vi "Optimal Angle Calc..vi"(8 "Command Angle":dbl, 9 "Feedback Angle":dbl, 11 "Speed":dbl) -> (0 "Angle":dbl, 3 "Speed":dbl)   [LabVIEW 2018]
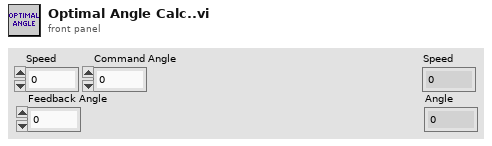
[diagram p1: front panel]
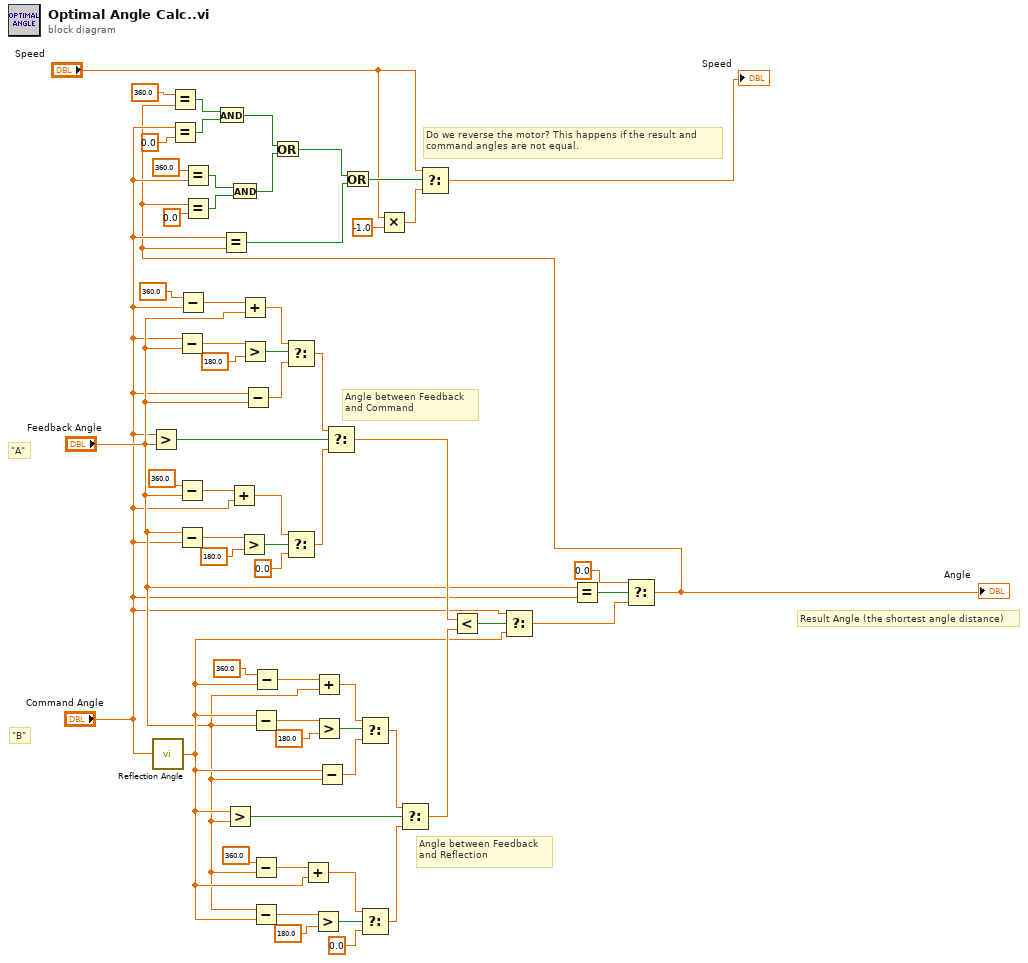
[diagram p0: block diagram]
diagram:
  # "Result Angle (the shortest angle distance)"
  # "Do we reverse the motor? This happens if the result and \ncommand angles are not equal."
  # "Angle between Feedback\nand Reflection"
  # "Angle between Feedback\nand Command"
  # "\"B\""
  # "\"A\""
  n1 = Greater?(x="Command Angle", y="Feedback Angle") -> (0:w61:bool)
  n2 = call "Reflection Angle.vi"("Command Angle"="Command Angle") -> ("Reflection Angle"=w24:dbl)  [unwired: 4 in]
  n3 = Equal?(x="Command Angle", y=0.0) -> (x = y?=w20:bool)
  n4 = Subtract(x="Command Angle", y="Feedback Angle") -> (x-y=w60:dbl)
  n5 = Subtract(x=360.0, y="Feedback Angle") -> (x-y=w48:dbl)
  n6 = Subtract(x="Feedback Angle", y="Command Angle") -> (x-y=w52:dbl)
  n7 = Subtract(x=360.0, y="Command Angle") -> (x-y=w56:dbl)
  n8 = Equal?(x=360.0, y="Command Angle") -> (x = y?=w18:bool)
  n9 = Greater?(x=w24, y="Feedback Angle") -> (0:w44:bool)
  n10 = Add(x=w48, y="Command Angle") -> (x+y=w47:dbl)
  n11 = Greater?(x=w52, y=180.0) -> (0:w50:bool)
  n12 = Add(x=w56, y="Feedback Angle") -> (x+y=w55:dbl)
  n13 = Greater?(x=w60, y=180.0) -> (0:w58:bool)
  n14 = Subtract(x="Command Angle", y="Feedback Angle") -> (x-y=w54:dbl)
  n15 = Subtract(x=w24, y="Feedback Angle") -> (x-y=w43:dbl)
  n16 = Subtract(x=360.0, y="Feedback Angle") -> (x-y=w31:dbl)
  n17 = Subtract(x="Feedback Angle", y=w24) -> (x-y=w35:dbl)
  n18 = Subtract(x=360.0, y=w24) -> (x-y=w39:dbl)
  n19 = Select(t=w55, s=w58, f=w54) -> (s? t:f=w53:dbl)
  n20 = Select(t=w47, s=w50, f=0.0) -> (s? t:f=w45:dbl)
  n21 = Add(x=w31, y=w24) -> (x+y=w30:dbl)
  n22 = Greater?(x=w35, y=180.0) -> (0:w33:bool)
  n23 = Add(x=w39, y="Feedback Angle") -> (x+y=w38:dbl)
  n24 = Greater?(x=w43, y=180.0) -> (0:w41:bool)
  n25 = Subtract(x=w24, y="Feedback Angle") -> (x-y=w37:dbl)
  n26 = Select(t=w53, s=w61, f=w45) -> (s? t:f=w27:dbl)
  n27 = Select(t=w38, s=w41, f=w37) -> (s? t:f=w36:dbl)
  n28 = Select(t=w30, s=w33, f=0.0) -> (s? t:f=w28:dbl)
  n29 = Multiply(x="Speed", y=-1.0) -> (x*y=w8:dbl)
  n30 = Select(t=w36, s=w44, f=w28) -> (s? t:f=w26:dbl)
  n31 = Less?(x=w27, y=w26) -> (x < y?=w25:bool)
  n32 = Select(t="Command Angle", s=w25, f=w24) -> (s? t:f=w2:dbl)
  n33 = Equal?(x="Feedback Angle", y="Command Angle") -> (x = y?=w4:bool)
  n34 = Select(t=0.0, s=w4, f=w2) -> (s? t:f=w1:dbl)
  "Angle" <- w1
  n35 = Equal?(x=360.0, y=w1) -> (x = y?=w21:bool)
  n36 = Equal?(x=w1, y=0.0) -> (x = y?=w17:bool)
  n37 = And(x=w21, y=w20) -> (x .and. y?=w15:bool)
  n38 = Equal?(x="Command Angle", y=w1) -> (x = y?=w13:bool)
  n39 = And(x=w18, y=w17) -> (x .and. y?=w14:bool)
  n40 = Or(x=w15, y=w14) -> (x .or. y?=w12:bool)
  n41 = Or(x=w12, y=w13) -> (x .or. y?=w11:bool)
  n42 = Select(t="Speed", s=w11, f=w8) -> (s? t:f=→"Speed":dbl)
